vi "LogFile.vi"(6 "File":path, 8 "Filename (optional)":string, 9 "Project Name (Unlimited length... Key word for analyzer, or folder for MIDAS settings file database)":string, 10 "Variable name (SAVE and LOAD are magic keywords for the MIDAS settings file database)":string, 11 "Category (SETTINGS_FILE is a magic keyword for the MIDAS settings file database)":string) -> (0 "MD5 Error out":errorcluster, 1 "Log This Error Out":errorcluster, 3 "MD5 message-digest":string)   [LabVIEW 2018, in "feGEM DataPacker.lvlib"]
uses:
  feGEM DataPacker.lvlib
  7c163460-8361-4dcd-911c-0cc4a201ad12.vi
  7c163460-8361-4dcd-911c-0cc4a201ad12.vi/d7e6c9b9-391b-4ab3-8a75-f8439391d001.vi
panel:
  out "string":string
  out "data":string
  out "length":i32
  out "size (in bytes)":i64
  out "size (in bytes) in memory":i32
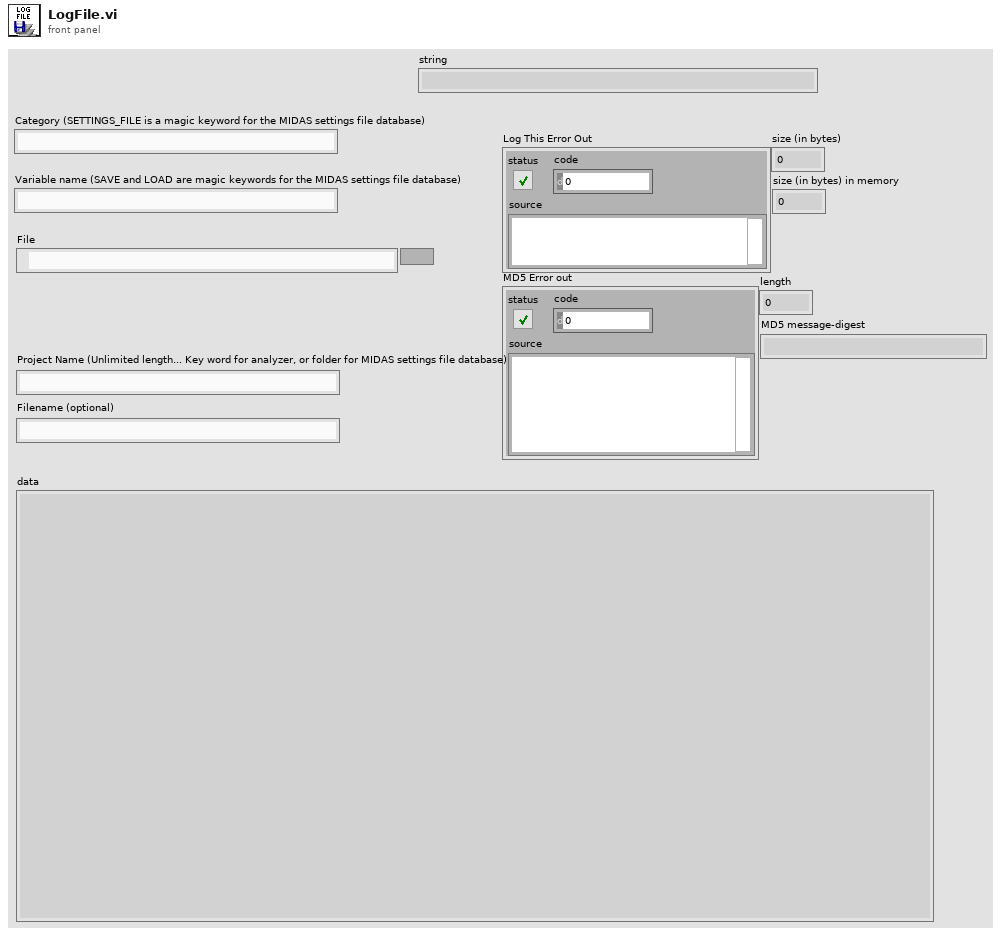
[diagram p1: front panel]
types:
  T1 = enum16{"open", "replace", "create", "open or create", "replace or create", "replace or create with confirmation"}
  T2 = enum16{"big-endian, network order", "native, host order", "little-endian"}
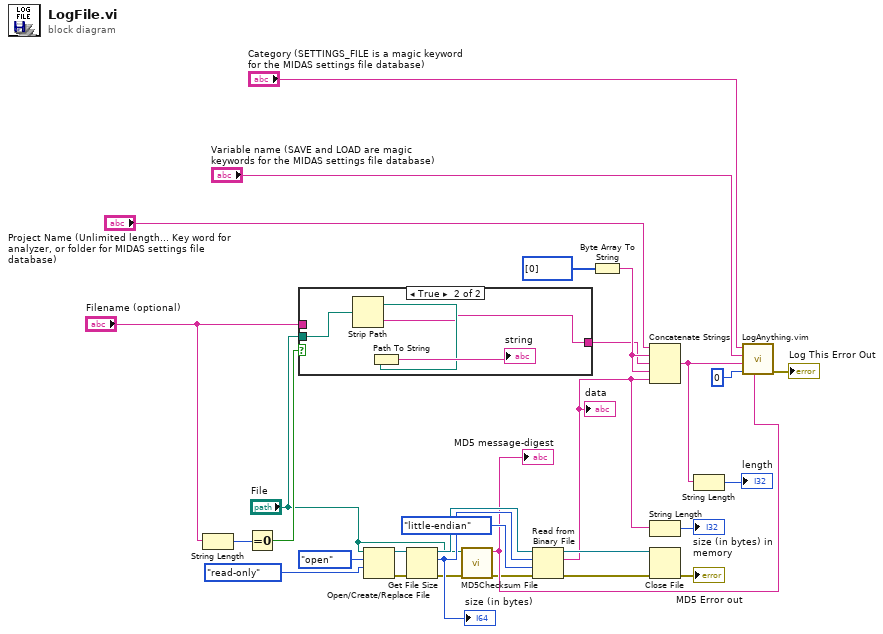
[diagram p0: block diagram]
diagram:
  n1 = String Length(string="Filename (optional)") -> (length=w5:i32)
  n2 = Equal To 0?(x=w5) -> (x = 0?=w4:bool)
  n3 = case shown="True" w4 {
    tunnel: [w30 w31] -> w3
    tunnel: "Filename (optional)" -> [w30 _]
    tunnel: "File" -> [_ w33]
    frame False {
    }
    frame True {
      n4 = Strip Path(path=w33) -> (stripped path=w32:path, name=w31:string)
      n5 = Path To String(path=w32) -> (string=→"string":string)
    }
  }
  n6 = Open/Create/Replace File(file path (use dialog)="File", operation (0:open)=T1."open", access (0:read/write)=enum16{"read/write", "read-only", "write-only"}."read-only") -> (refnum out=w14:refnum<file>, error out=w12:errorcluster)  [unwired: 3 in, 1 out]
  n7 = Get File Size(file=w14, error in=w12) -> (refnum out=w13:refnum<file>, size (in bytes)=w11:i64, 0:w7:errorcluster)
  "size (in bytes)" <- w11
  n8 = call <vilib>:"MD5Checksum File.vi"("error in (no error)"=w7, "Path"="File") -> ("error out"=w6:errorcluster, "MD5 message-digest"=w8:string)  [unwired: 8 in]
  "MD5 message-digest" <- w8
  n9 = Read from Binary File(8:w6, 9:T2."little-endian" ("byte order (0:big-endian, network order)"), 10:w11, 11:w13) -> (0:w15:errorcluster, 2:w10:string, 3:w16:refnum<file>)  [unwired: 2 in, 1 out]
  "data" <- w10
  n10 = Byte Array To String(unsigned byte array=u8[] [0]) -> (string=w25:string)
  n11 = Concatenate Strings("Project Name (Unlimited length... Key word for analyzer, or folder for MIDAS settings file database)", w25, w3, w25, w10) -> (w18:string)
  n12 = String Length(string=w10) -> (length=→"size (in bytes) in memory":i32)
  n13 = Close File(refnum=w16, error in=w15) -> (error out=→"MD5 Error out":errorcluster)  [unwired: 1 out]
  n14 = String Length(string=w18) -> (length=→"length":i32)
  n15 = call "LogAnything.vim"("Equipment description (32 chars)"=w8, "Period to update history plots (seconds)\nUnset (65535) = Use MIDAS default in ODB\n0 = Record but do not put in histories"=u16 0 ("Period to update history plots (seconds)\nUnset (65535) = Use MIDAS default in ODB\n0 = Record but do not put in histories"), "Array"=w18, "Variable Name"="Variable name (SAVE and LOAD are magic keywords for the MIDAS settings file database)", "Category"="Category (SETTINGS_FILE is a magic keyword for the MIDAS settings file database)") -> ("error out"=→"Log This Error Out":errorcluster)  [unwired: 6 in]
